vi "ApplyPropertyTemplateToMethod.vi"(0 "ClassWriterGOOP300 in":refnum<class "ClassWriterGOOP300.lvclass">, 1 "VIRef":refnum<vi>, 2 "ClassRef":refnum<vi>, 3 "PropertyName":string, 4 "MethodTemplateName":string, 5 "error in (no error)":errorcluster) -> (14 "ClassWriterGOOP300 out":refnum<class "ClassWriterGOOP300.lvclass">, 19 "error out":errorcluster)   [LabVIEW 2020, in "ClassWriterGOOP300.lvclass"]
uses:
  <resource>/Framework/Providers/Open_GDS/ClassProviders/Provider_EndevoGOOP300/ClassWriterGOOP300_class/ClassWriterGOOP300.lvclass
  <resource>/Framework/Providers/Open_GDS/ClassProviders/Provider_LvNativeClass/ClassWriterNative_class/ClassWriterNative.lvclass
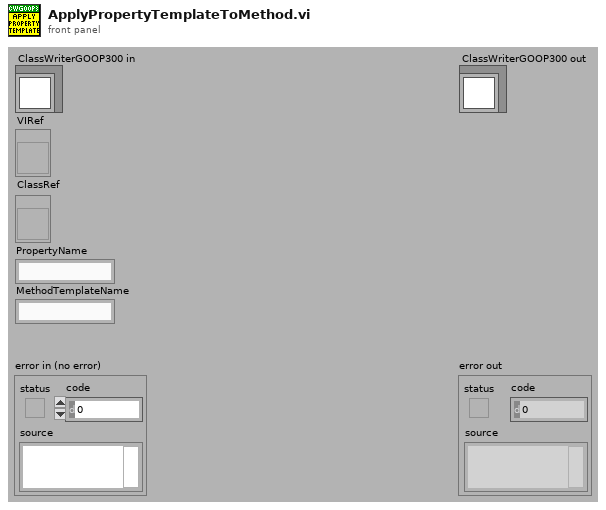
[diagram p1: front panel]
types:
  T1 = enum32{"Bad", "Idle", "Run top level", "Running"}
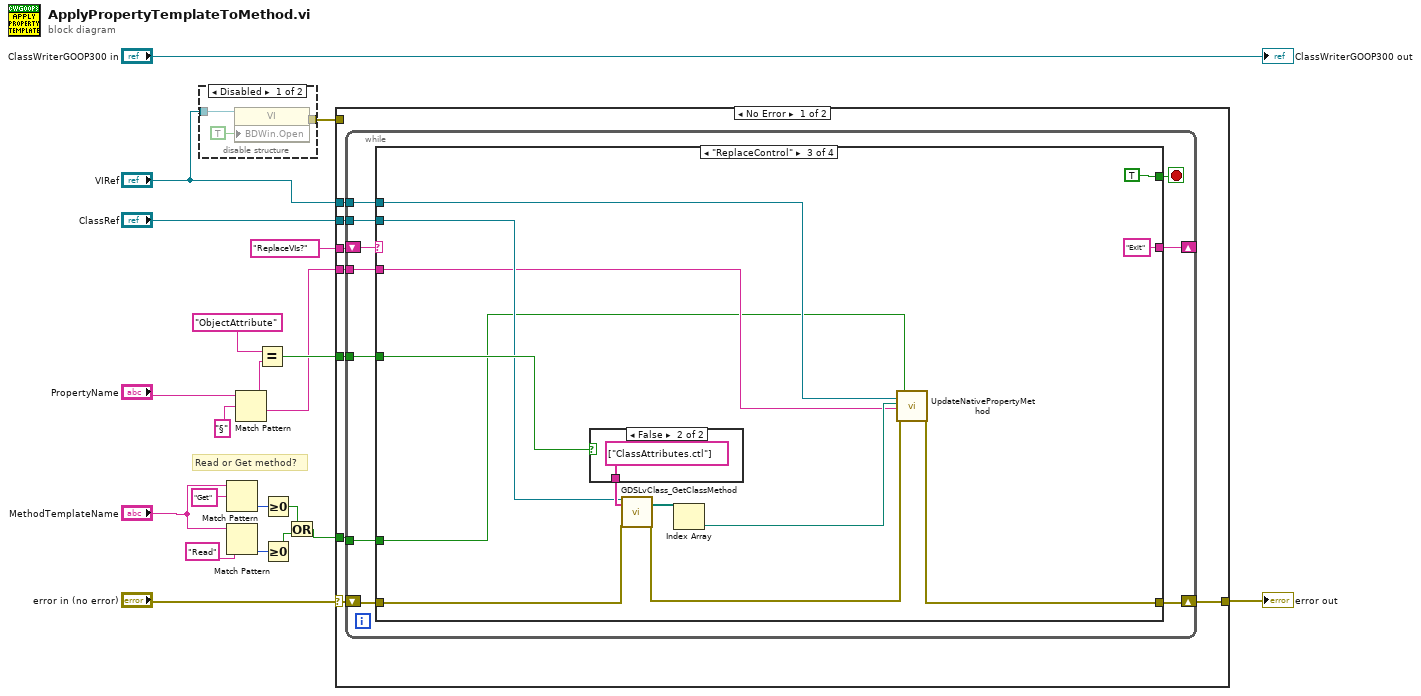
[diagram p0: block diagram]
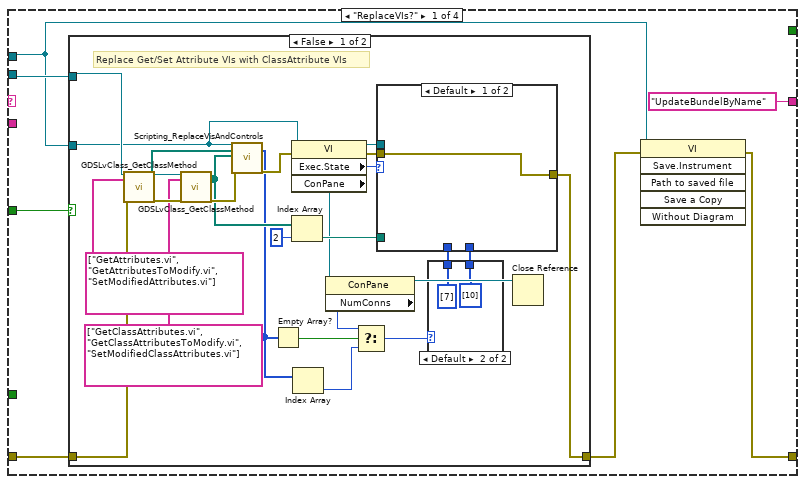
[diagram p3: hidden frame]
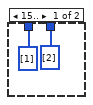
[diagram p4: hidden frame]
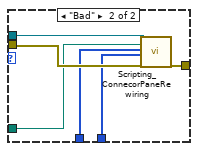
[diagram p5: hidden frame]
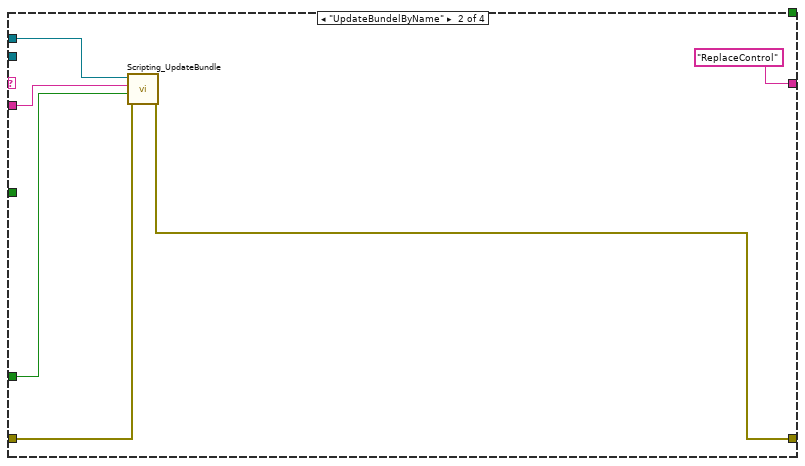
[diagram p7: hidden frame]
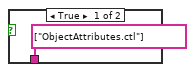
[diagram p8: hidden frame]
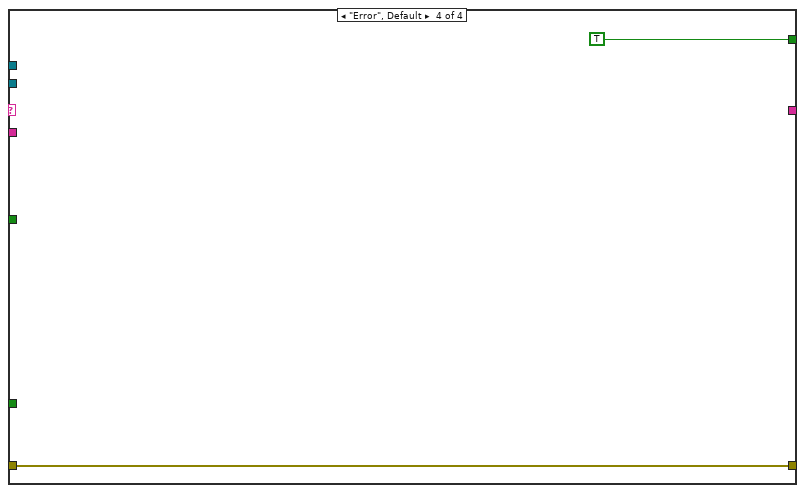
[diagram p9: hidden frame]
diagram:
  # "Read or Get method?"
  n1 = disable-structure shown="Disabled" {
    disable-tunnel: "VIRef" -> [w23 _]
    disable-tunnel: [w22 _] -> w1
    frame Disabled {
      n2 = property class="VI"(reference=w23, "BDWin.Open"=TRUE ("Block Diagram Window:Open")) -> (error out=w22:errorcluster)  [unwired: 1 in, 1 out]
    }
    frame Enabled {
    }
  }
  n3 = Match Pattern(string="MethodTemplateName", regular expression="Get") -> (offset past match=w7:i32)  [unwired: 1 in, 3 out]
  n4 = Match Pattern(string="MethodTemplateName", regular expression="Read") -> (offset past match=w9:i32)  [unwired: 1 in, 3 out]
  n5 = Match Pattern(string="PropertyName", regular expression="§" ("search string")) -> (before substring=w19:string, after substring=w16:string)  [unwired: 1 in, 2 out]
  n6 = Equal?(x="ObjectAttribute" ("string"), y=w19) -> (x = y?=w17:bool)
  n7 = Greater Or Equal To 0?(x=w7) -> (x >= 0?=w5:bool)
  n8 = Greater Or Equal To 0?(x=w9) -> (x >= 0?=w6:bool)
  n9 = Or(x=w5, y=w6) -> (x .or. y?=w3:bool)
  n10 = case shown="No Error" "error in (no error)" {
    selector: "error in (no error)" -> [w26 w111]
    tunnel: "ReplaceVIs?" -> [w32 _]
    tunnel: "VIRef" -> [w31 _]
    tunnel: "ClassRef" -> [w30 _]
    tunnel: w3 -> [w29 _]
    tunnel: w16 -> [w28 _]
    tunnel: [w27 w111] -> w11
    tunnel: w17 -> [w25 _]
    tunnel: w1 -> [_ _]
    frame No Error {
      n11 = while {
        tunnel: w31 -> [w42]
        tunnel: w28 -> [w41]
        shift-right: [w39] -> w27
        shift-left: w26 -> [w40]
        shift-right: [w37] -> _
        shift-left: w32 -> [w38]
        tunnel: w30 -> [w35]
        tunnel: w29 -> [w34]
        tunnel: w25 -> [w33]
        stop <- w36 stop-if-true
        n12 = case shown="\"ReplaceControl\"" w38 {
          tunnel: w42 -> [w44 w92 w95 _]
          tunnel: w41 -> [_ w91 w96 _]
          tunnel: w40 -> [w47 w90 w98 w109]
          tunnel: [w45 w88 w97 w109] -> w39
          tunnel: ["UpdateBundelByName" "ReplaceControl" "Exit" _] -> w37
          tunnel: [_ _ TRUE TRUE] -> w36
          tunnel: w35 -> [w48 _ w100 _]
          tunnel: w34 -> [_ w89 w94 _]
          tunnel: w33 -> [w43 _ w101 _]
          frame "ReplaceVIs?" {
            n13 = case shown="False" w43 {
              tunnel: w48 -> [w74 _]
              tunnel: w44 -> [w67 _]
              tunnel: w47 -> [w73 w87]
              tunnel: [w62 w87] -> w46
              frame False {
                # "Replace Get/Set Attribute VIs with ClassAttribute VIs"
                n14 = call <resource>:"GDSLvClass_GetClassMethod.vi"("Class Refnum In"=w74, "VINames"=string[] ["GetAttributes.vi", "GetAttributesToModify.vi", "SetModifiedAttributes.vi"], "error in (no error)"=w73) -> ("Class Refnum Out"=w72:refnum<vi>, "ViPaths"=w68:path[], "error out"=w71:errorcluster)  [unwired: 13 in, 1 out]
                n15 = call <resource>:"GDSLvClass_GetClassMethod.vi"("Class Refnum In"=w72, "VINames"=string[] ["GetClassAttributes.vi", "GetClassAttributesToModify.vi", "SetModifiedClassAttributes.vi"], "error in (no error)"=w71) -> ("ViPaths"=w61:path[], "error out"=w70:errorcluster)  [unwired: 13 in, 2 out]
                n16 = call <resource>:"Scripting_ReplaceVisAndControls.vi"("ViRef"=w67, "OldVIsAndControls"=w68, "NewVIsAndControls"=w61, "error in (no error)"=w70) -> ("ReplacedVIsConPaneSize"=w51:u32[], "error out"=w63:errorcluster)  [unwired: 14 in]
                n17 = Empty Array?(array=w51) -> (empty?=w54:bool)
                n18 = property class="VI"(reference=w67, error in=w63) -> (reference out=w64:refnum<vi>, error out=w65:errorcluster, "Exec.State"=w66:T1, "ConPane"=w58:refnum<vi>)
                n19 = Index Array(array=w61, index=2) -> (element=w59:path)
                n20 = Index Array(array=w51) -> (element=w50:u32)  [unwired: 1 in]
                n21 = property class="ConPane"(reference=w58) -> (reference out=w57:refnum<vi>, "NumConns"=w53:u32)  [unwired: 1 in, 1 out]
                n22 = Select(t=w53, s=w54, f=w50) -> (s? t:f=w52:u32)
                n23 = case shown="Default" w52 {
                  tunnel: [u32[] [1] ("OldConnectorPaneIndex") u32[] [7] ("OldConnectorPaneIndex")] -> w56
                  tunnel: [u32[] [2] ("OldConnectorPaneIndex") u32[] [10] ("OldConnectorPaneIndex")] -> w55
                  frame 15.. {
                  }
                  frame Default {
                  }
                }
                n24 = case shown="Default" w66 {
                  tunnel: w65 -> [w80 w85]
                  tunnel: w64 -> [_ w86]
                  tunnel: [w80 w84] -> w62
                  tunnel: w59 -> [_ w83]
                  tunnel: w56 -> [_ w82]
                  tunnel: w55 -> [_ w81]
                  frame Default {
                  }
                  frame "Bad" {
                    n25 = call <resource>:"Scripting_ConnecorPaneRewiring.vi"("ViRef"=w86, "SubViThatHasChangedConnectorPane"=w83, "OldConnectorPaneIndex"=w82, "NewConnectorPaneIndex"=w81, "error in (no error)"=w85) -> ("error out"=w84:errorcluster)  [unwired: 14 in]
                  }
                }
                n26 = Close Reference(reference=w57) -> ()  [unwired: 1 in, 1 out]
              }
              frame True {
              }
            }
            n27 = invoke class="VI" method="Save.Instrument"(reference=w44, error in=w46) -> (error out=w45:errorcluster)  [unwired: 4 in, 5 out]
          }
          frame "UpdateBundelByName" {
            n28 = call <resource>:"Scripting_UpdateBundle.vi"("error in (no error)"=w90, "Boolean"=w89, "PropertyName"=w91, "VI in"=w92) -> ("error out"=w88:errorcluster)  [unwired: 7 in]
          }
          frame "ReplaceControl" {
            n29 = case shown="False" w101 {
              tunnel: [string[] ["ObjectAttributes.ctl"] ("VINames") string[] ["ClassAttributes.ctl"] ("VINames")] -> w103
              frame True {
              }
              frame False {
              }
            }
            n30 = call <resource>:"GDSLvClass_GetClassMethod.vi"("Class Refnum In"=w100, "VINames"=w103, "error in (no error)"=w98) -> ("ViPaths"=w104:path[], "error out"=w99:errorcluster)  [unwired: 13 in, 2 out]
            n31 = Index Array(array=w104) -> (element=w102:path)  [unwired: 1 in]
            n32 = call <resource>:"UpdateNativePropertyMethod.vi"("VI"=w95, "TypeDefControl"=w102, "Property"=w96, "error IO"=w99, "GetMethod"=w94) -> ("error out"=w97:errorcluster)  [unwired: 14 in]
          }
          frame "Error", Default {
          }
        }
      }
    }
    frame Error {
    }
  }
  "error out" <- w11
  "ClassWriterGOOP300 out" <- "ClassWriterGOOP300 in"
